vi "Get TDMS Content.vi"(8 "Error In":errorcluster, 11 "File Path Control":path) -> (0 "Error Out":errorcluster, 3 "Channel selector":T1[](array[typedef]))   [LabVIEW 2018]
uses:
  Controls/NXG TDMS channel selector entry.ctl
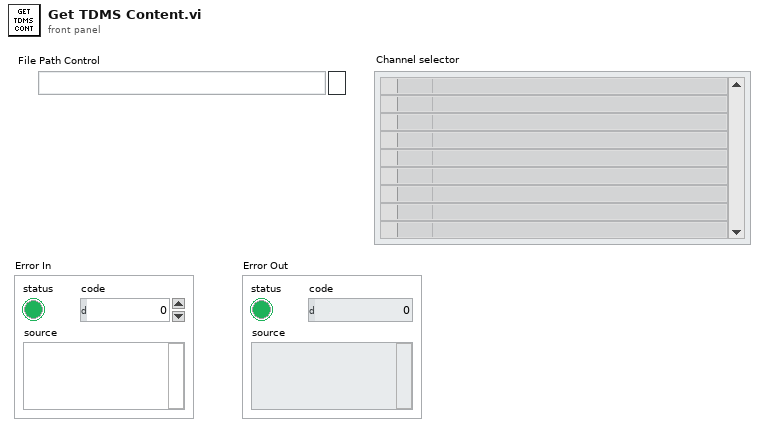
[diagram p1: front panel]
types:
  T1 = typedef "NXG TDMS channel selector entry.ctl" = cluster{"Group":string, "Channel":string, "Active":bool}
  T2 = typedef "File_Group_Chan_Abbr.ctl" = cluster{"File Path Control":path, "Group":string, "Channel":string, "Abbreviated":string}
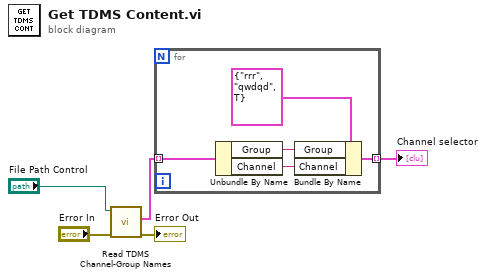
[diagram p0: block diagram]
diagram:
  n1 = call "Read TDMS Channel-Group Names.vi"("error in"="Error In", "File Path Control"="File Path Control") -> ("error out"=→"Error Out":errorcluster, "File-group-channel"=w4:T2[])  [unwired: 8 in]
  n2 = for {
    tunnel: w4 -> [w9] mode=indexing
    tunnel: [w6] -> w3 mode=indexing
    n3 = Unbundle By Name(w9) -> ("Group"=w8:string, "Channel"=w7:string)
    n4 = Bundle By Name(cluster=T1 {"Group"="rrr", "Channel"="qwdqd", "Active"=TRUE} ("Cluster"), "Group"=w8, "Channel"=w7) -> (w6:T1)
  }
  "Channel selector" <- w3
